vi "Set Baud Rate Values.vi"(9 "PID":string, 10 "Channel Index":i32, 11 "Channel Str":string[](array[string])) -> (3 "Baud Rate Strings And Values":T1)   [LabVIEW 2021]
uses:
  <vilib>/Utility/miscctls.llb/LVStringsAndValuesArrayTypeDef_U32.ctl
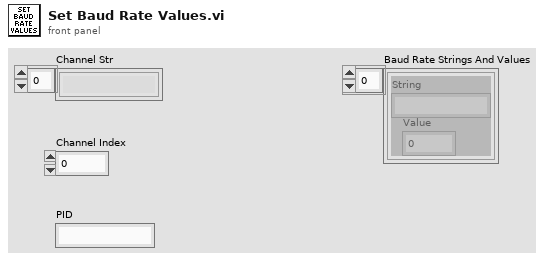
[diagram p1: front panel]
types:
  T1 = typedef "LVStringsAndValuesArrayTypeDef_U32.ctl" = cluster{"String":string, "Value":u32}[]
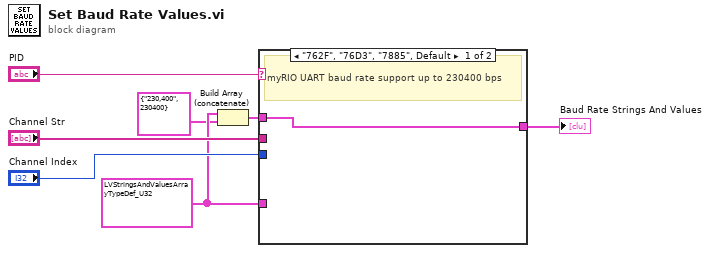
[diagram p0: block diagram]
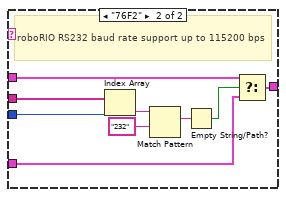
[diagram p2: hidden frame]
diagram:
  w3 = T1 [{"String"="110", "Value"=110}, {"String"="300", "Value"=300}, {"String"="600", "Value"=600}, {"String"="1,200", "Value"=1200}, {"String"="2,400", "Value"=2400}, {"String"="4,800", "Value"=4800}, {"String"="9,600", "Value"=9600}, {"String"="19,200", "Value"=19200}, {"String"="38,400", "Value"=38400}, {"String"="57,600", "Value"=57600}, {"String"="115,200", "Value"=115200}] ("Strings And Values []")
  n1 = Build Array (concatenate)(w3, cluster{"String":string, "Value":u32} {"String"="230,400", "Value"=230400}) -> (w1:T1)
  n2 = case shown="\"762F\", \"76D3\", \"7885\", Default" "PID" {
    tunnel: [w8 w17] -> w4
    tunnel: w1 -> [w8 w16]
    tunnel: w3 -> [_ w15]
    tunnel: "Channel Str" -> [_ w10]
    tunnel: "Channel Index" -> [_ w9]
    frame "762F", "76D3", "7885", Default {
      # "myRIO UART baud rate support up to 230400 bps"
    }
    frame "76F2" {
      # "roboRIO RS232 baud rate support up to 115200 bps"
      n3 = Index Array(array=w10, index=w9) -> (element=w12:string)
      n4 = Match Pattern(string=w12, regular expression="232") -> (match substring=w14:string)  [unwired: 1 in, 3 out]
      n5 = Empty String/Path?(string/path=w14) -> (empty?=w11:bool)
      n6 = Select(t=w16, s=w11, f=w15) -> (s? t:f=w17:T1)
    }
  }
  "Baud Rate Strings And Values" <- w4
